vi "HL Grab.vi"() -> ()   [LabVIEW 2014]
doc: "The HL Grab VI acquires images continuously and displays the images in an image control using high-level acquisition VIs. A grab is appropriate for high-speed applications that process only one image at a time."
panel:
  out "Frame Rate":dbl(knob) scale=0.0..100.0
  out "Image":T1(plugin-control)
  in  "Interface Name":string="img0"
  in  "Stop":bool
  # "Overview: Demonstrates how to perform acquires images continuously and displays the images in an image control using high-level acquisition VIs. \nRequirements: Vision Acquisition Software, IMAQ frame grabber.\nInstructions: \n1. Select the IMAQ frame grabber Interface Name.\n2. Run the VI."
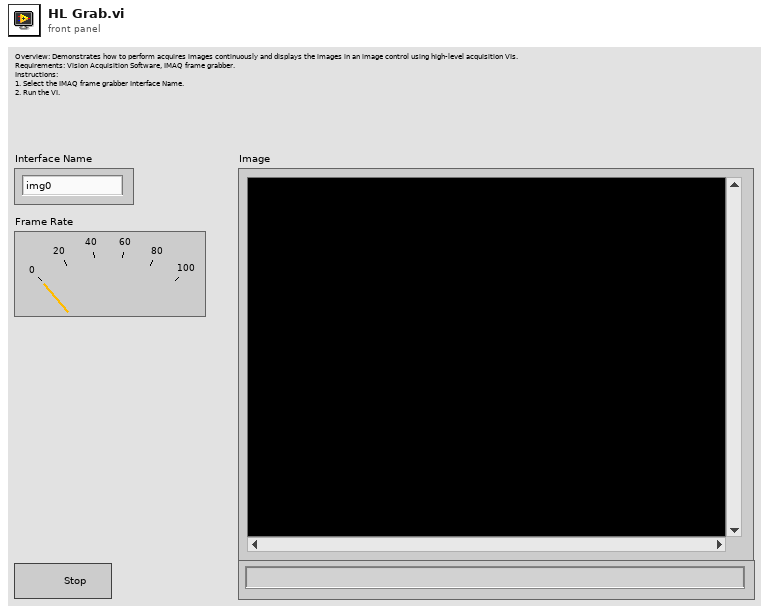
[diagram p1: front panel]
types:
  T1 = typedef "IMAQ Image.ctl" = refnum<image>
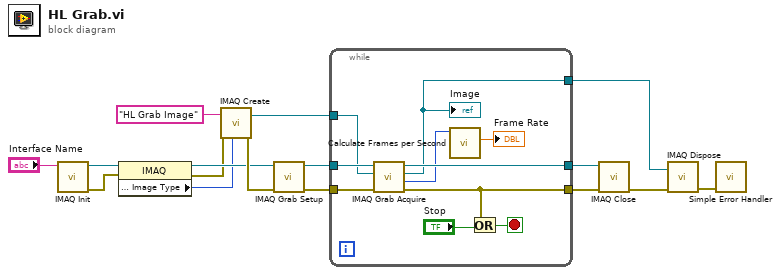
[diagram p0: block diagram]
diagram:
  n1 = call <vilib>:"IMAQ Init.vi"("Interface Name"="Interface Name") -> ("error out"=w8:errorcluster, "IMAQ Session Out"=w9:refnum<k11>)  [unwired: 1 in, 8 out]
  n2 = property class="IMAQ"(reference=w9, error in=w8) -> (reference out=w7:refnum<k11>, error out=w6:errorcluster, "Image Parameters : Image Type"=w5:u32)
  n3 = call "IMAQ Create"("Image Name"="HL Grab Image", "Image Type"=w5, "error in (no error)"=w6) -> ("New Image"=w15:T1, "error out"=w16:errorcluster)  [unwired: 1 in, 1 out]
  n4 = call <vilib>:"IMAQ Grab Setup.vi"("error in (no error)"=w16, "IMAQ Session In"=w7) -> ("error out"=w13:errorcluster, "IMAQ Session Out"=w14:refnum<k11>)  [unwired: 8 out]
  n5 = while {
    tunnel: [w21] -> w10
    tunnel: w15 -> [w24]
    tunnel: w14 -> [w25]
    tunnel: w13 -> [w26]
    tunnel: [w19] -> w4
    tunnel: [w20] -> w2
    stop <- w23 stop-if-true
    n6 = call <vilib>:"IMAQ Grab Acquire.vi"("error in (no error)"=w26, "Image In"=w24, "IMAQ Session In"=w25) -> ("error out"=w19:errorcluster, "Acquired Buffer Number"=w18:u32, "Image Out"=w20:T1, "IMAQ Session Out"=w21:refnum<k11>)  [unwired: 1 in, 4 out]
    "Image" <- w20
    n7 = call <vilib>:"Calculate Frames per Second.vi"("Buffer Number"=w18) -> ("Processed Frames/s"=→"Frame Rate":dbl)  [unwired: 8 in, 2 out]
    n8 = Or(x=w19, y="Stop") -> (x .or. y?=w23:bool)
  }
  n9 = call <vilib>:"IMAQ Close.vi"("error in (no error)"=w4, "IMAQ Session In"=w10) -> ("error out"=w3:errorcluster)  [unwired: 9 out]
  n10 = call "IMAQ Dispose"("Image"=w2, "error in (no error)"=w3) -> ("error out"=w1:errorcluster)  [unwired: 1 in, 3 out]
  n11 = call <vilib>:"Simple Error Handler.vi"("error in (no error)"=w1) -> ()  [unwired: 1 in, 8 out]
